vi "User Console.vi"(8 "error in":errorcluster) -> (0 "error out":errorcluster)   [LabVIEW 2020]
doc: "User Console thread VI"
uses:
  Controls/Events_User.ctl
  Database/Controls/Account Database.ctl
  Controls/Data_Initialize.ctl
  SubVIs/User Event - Stop/User Event - Stop.lvlib
  <vilib>/Utility/error.llb/Error Cluster From Error Code.vi
  <vilib>/ErrorRing/Error Ring.xnode
  SubVIs/Message Queue/Message Queue.lvlib
  SubVIs/Message Queue/Enqueue Message (Single).vi
  FGV/Controls/FGV_State.ctl
  Controls/User Console references.ctl
  Controls/User console Local Data.ctl
  Controls/Keypad.ctl
  Controls/Transactions.ctl
  Controls/User Console.ctl
panel:
  in  "User Console":T1
  # "[Covers: UI2]"
  # "[Covers: UI1]"
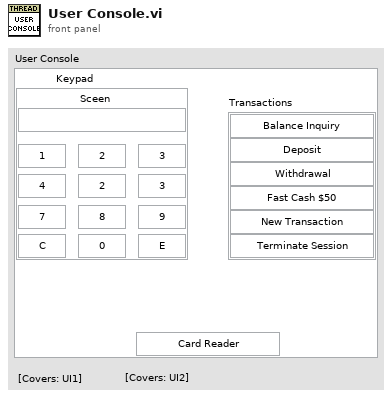
[diagram p1: front panel]
types:
  T1 = typedef "User Console.ctl" = cluster{"Keypad":T2, "Transactions":T3, "Card Reader":bool}
  T2 = typedef "Keypad.ctl" = cluster{"Sceen":string, "1":bool, "2":bool, "3":bool, "4":bool, "5":bool, "6":bool, "7":bool, "8":bool, "9":bool, "C":bool, "0":bool, "E":bool}
  T3 = typedef "Transactions.ctl" = cluster{"Balance Inquiry":bool, "Deposit":bool, "Withdrawal":bool, "Fast Cash $50":bool, "New Transaction":bool, "Terminate Session":bool}
  T4 = enum32{"Invalid", "Standard", "Closed", "Hidden", "Minimized", "Maximized"}
  T5 = typedef "FGV_State.ctl" = enum16{"1 - OpenDatabase", "2 - Initialize Events", "3 - Initialize QMH", "4 - Close QMH", "5 - Close Events", "Read FGV", "Save Database", "Def"}
  T6 = typedef "FGV_Data.ctl" = cluster{"QMH":T7, "User Events":T8, "Database":T9[]}
  T7 = typedef "Message Queue.lvlib/All Message Queues.ctl" = cluster{"User Console":refnum<queue>, "Display Console":refnum<queue>, "Sensor Interface":refnum<queue>, "Process":refnum<queue>}
  T8 = typedef "Events_User.ctl" = cluster{"Stop User Console":refnum<user-event>, "Error User Console":refnum<user-event>, "Stop Sensor Interface ":refnum<user-event>, "Error Sensor Interface":refnum<user-event>}
  T9 = typedef "Account Database.ctl" = cluster{"Account Number":i32, "First Name":string, "Last Name":string, "Balance":dbl}
  T10 = typedef "User console Local Data.ctl" = cluster{"Initiliaze":T11, "User Console Ref":T12, "Configuration Database":T9}
  T11 = typedef "Data_Initialize.ctl" = cluster{"Database":T9[], "User Events":T8}
  T12 = typedef "User Console references.ctl" = cluster{"0":refnum<vi>, "1":refnum<vi>, "2":refnum<vi>, "3":refnum<vi>, "4":refnum<vi>, "5":refnum<vi>, "6":refnum<vi>, "7":refnum<vi>, "8":refnum<vi>, "9":refnum<vi>, "Deposit":refnum<vi>, "Fast Cash $50":refnum<vi>, "Balance Inquiry":refnum<vi>, "Sceen":refnum<vi>, "Card Reader":refnum<vi>, "Withdrawal":refnum<vi>, "New Transaction":refnum<vi>, "Terminate Session":refnum<vi>, "E":refnum<vi>, "C":refnum<vi>}
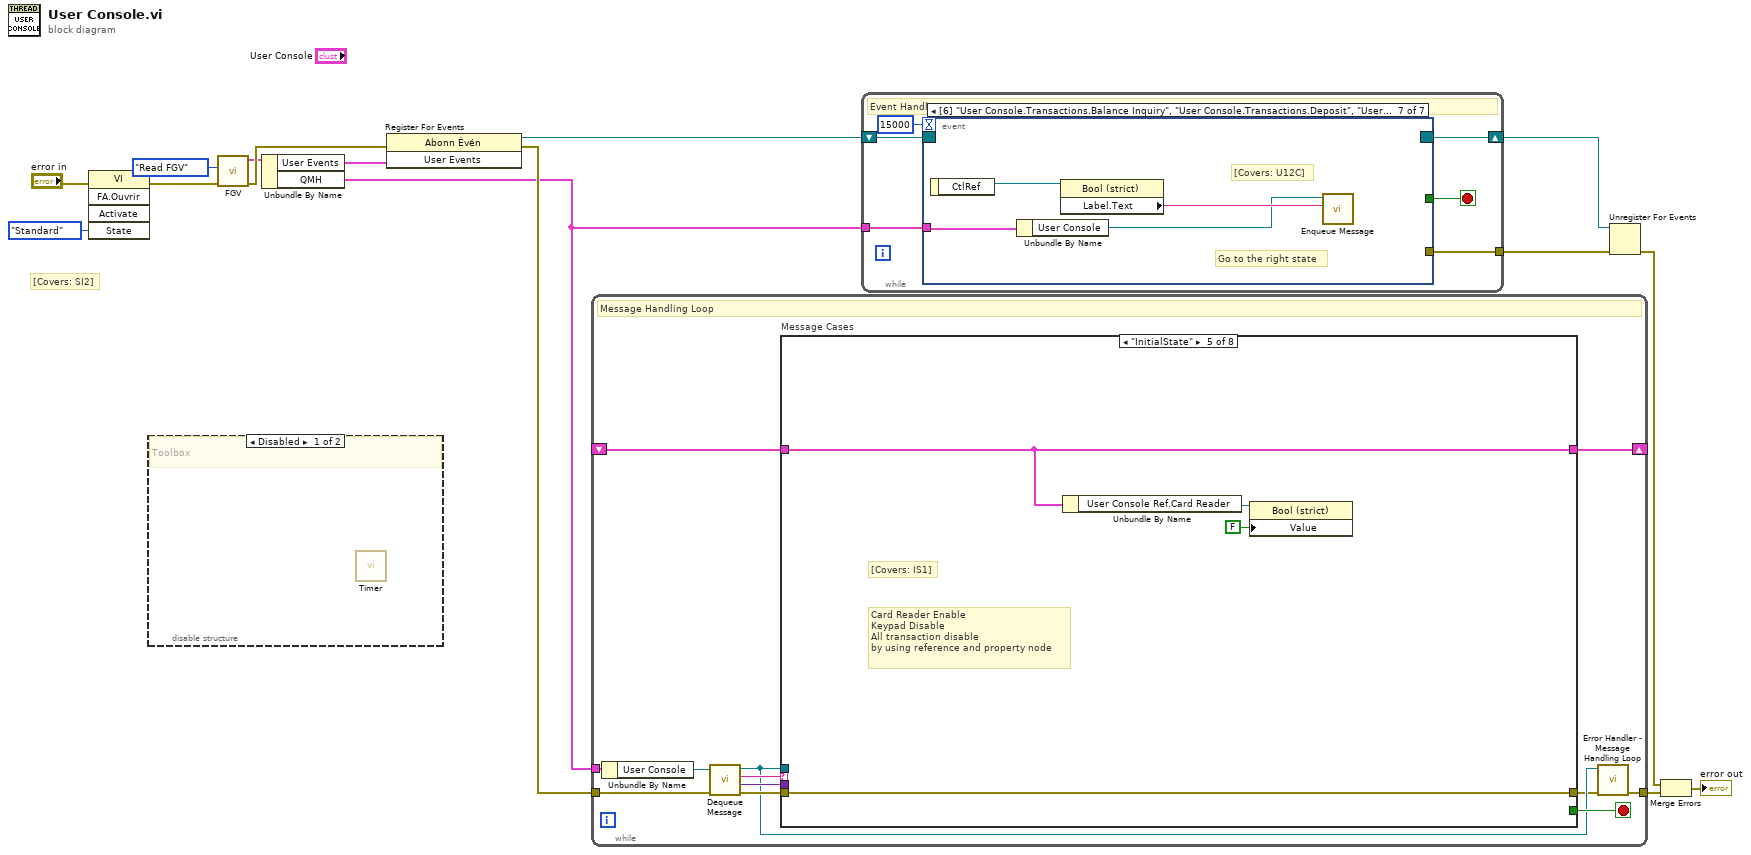
[diagram p0: block diagram]
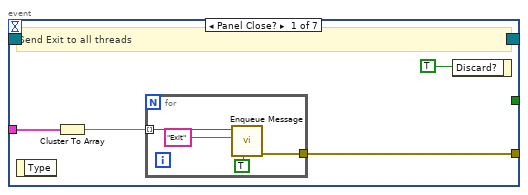
[diagram p3: hidden frame]
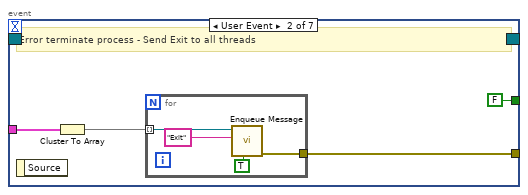
[diagram p4: hidden frame]
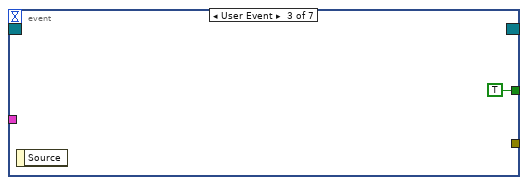
[diagram p5: hidden frame]
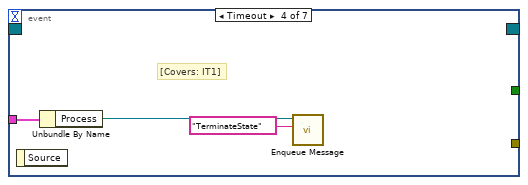
[diagram p6: hidden frame]
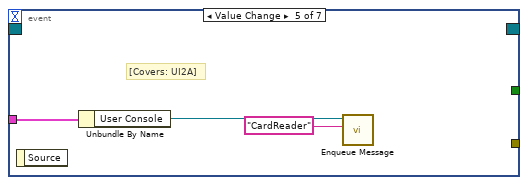
[diagram p7: hidden frame]
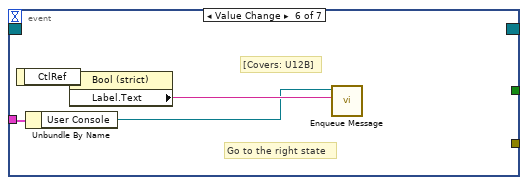
[diagram p8: hidden frame]
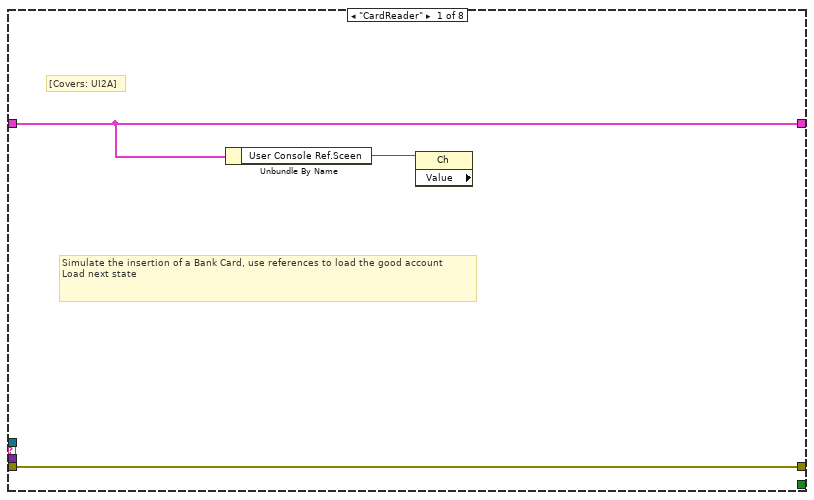
[diagram p9: hidden frame]
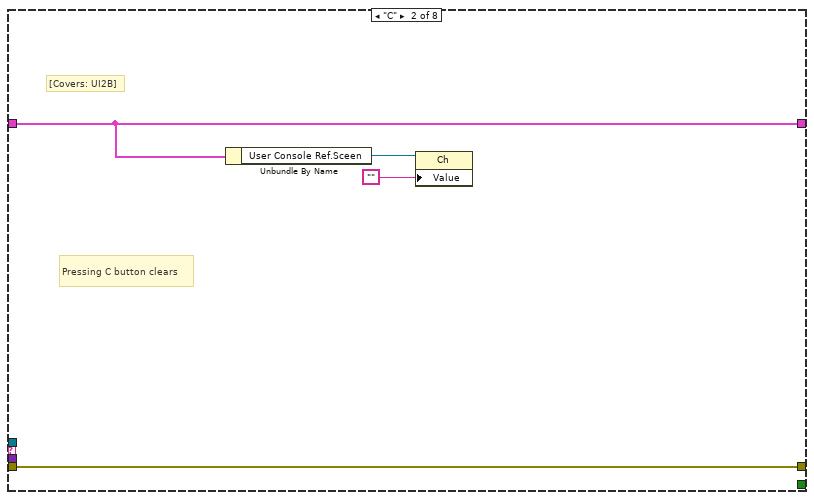
[diagram p10: hidden frame]
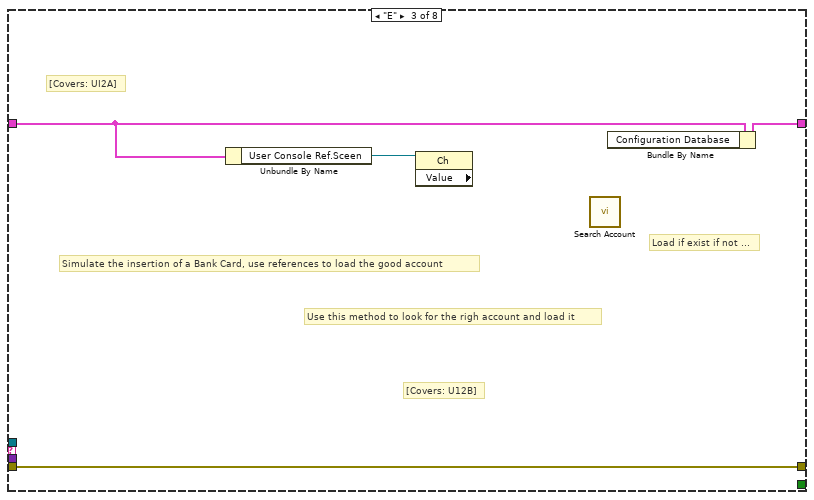
[diagram p11: hidden frame]
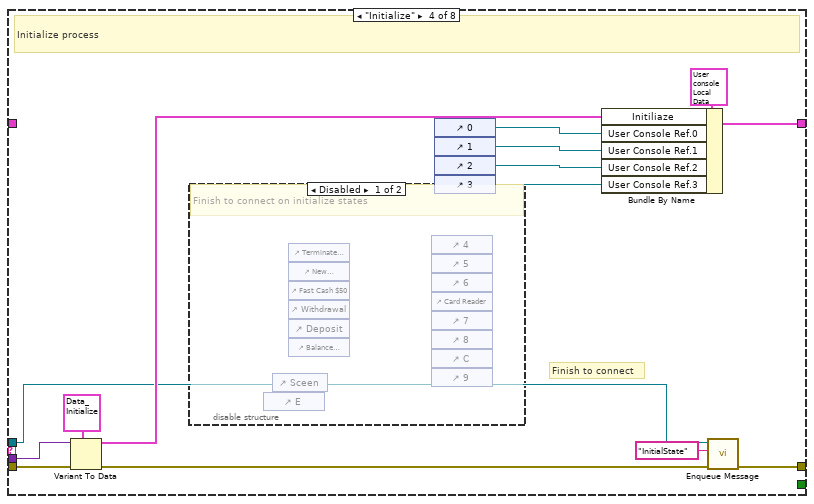
[diagram p12: hidden frame]
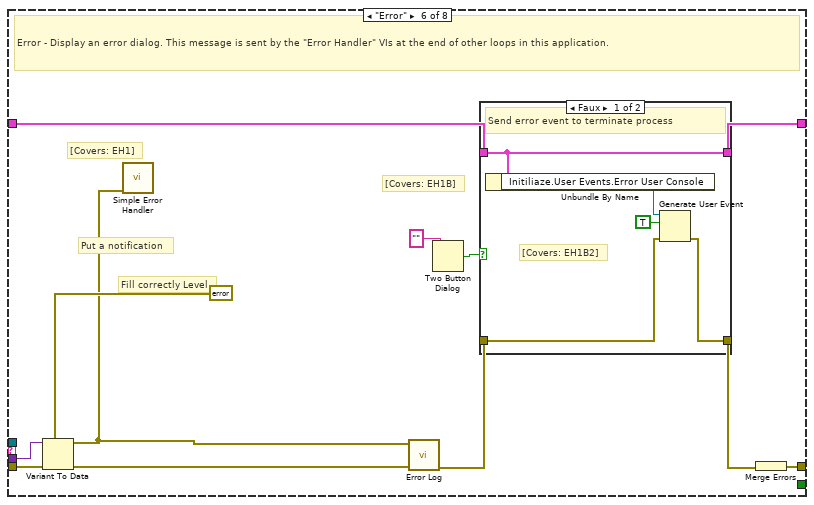
[diagram p14: hidden frame]
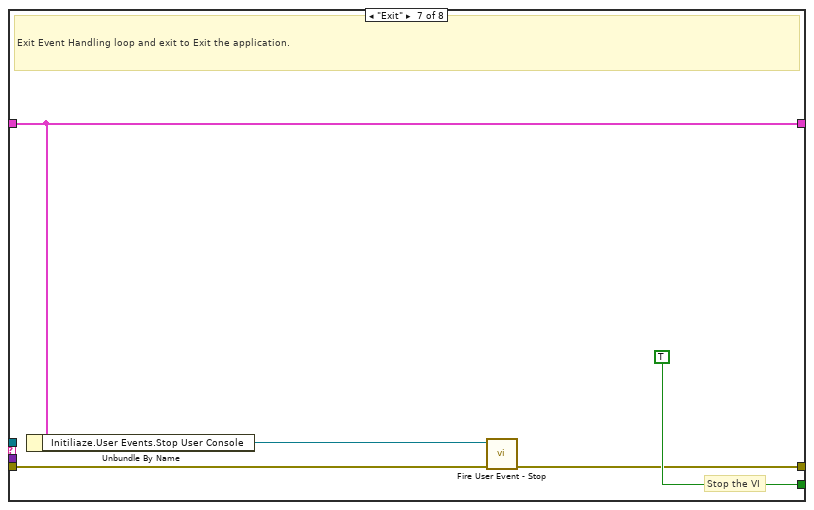
[diagram p16: hidden frame]
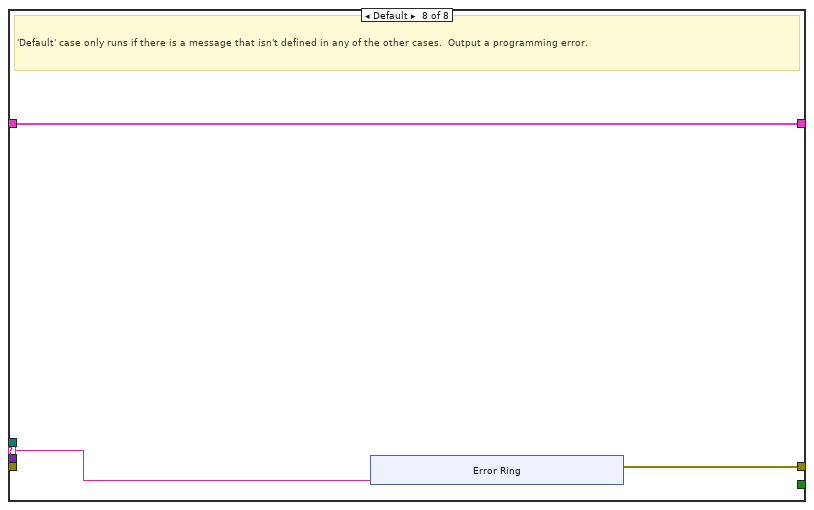
[diagram p17: hidden frame]
diagram:
  # "[Covers: SI2]"
  n1 = invoke class="VI" method="FA.Ouvrir"(error in="error in", "State"=T4."Standard") -> (error out=w2:errorcluster)  [unwired: 3 in, 4 out]
  n2 = disable-structure shown="Disabled" {
    frame Disabled {
      # "Toolbox"
      n3 = call "Timer.vi"() -> ()  [unwired: 9 in, 3 out]
    }
    frame Enabled {
    }
  }
  n4 = call "FGV.vi"("error in (no error)"=w2, "FGV_State"=FGV_State."Read FGV") -> ("error out"=w12:errorcluster, "FGV 2"=w10:T6)  [unwired: 8 in]
  n5 = Unbundle By Name(w10) -> ("User Events"=w11:T8, "QMH"=w14:T7)
  n6 = register-events(error in=w12, w11) -> (reference out=w8:refnum<event-registration>, error out=w15:errorcluster)  [unwired: 1 in]
  n7 = while {
    tunnel: w14 -> [w17]
    shift-right: [w26] -> _
    shift-left: _ -> [w27]
    tunnel: w15 -> [w24]
    tunnel: [w19] -> w4
    stop <- w25 stop-if-true
    # "Message Handling Loop"
    n8 = Unbundle By Name(w17) -> ("User Console"=w16:refnum<queue>)
    n9 = call "Dequeue Message.vi"("error in (no error)"=w24, "Message Queue"=w16) -> ("error out"=w23:errorcluster, "Message Data"=w21:variant, "Message"=w22:string, "dup Message Queue"=w20:refnum<queue>)  [unwired: 6 in]
    n10 = case "Message Cases" shown="\"InitialState\"" w22 {
      selector: w22 -> [_ _ _ _ _ _ _ w81]
      tunnel: w20 -> [_ _ _ w40 _ _ _ _]
      tunnel: w23 -> [w30 w34 w38 w51 w56 w68 w77 _]
      tunnel: [w30 w34 w38 w39 w56 w65 w76 w82] -> w18
      tunnel: w27 -> [w28 w32 w37 _ w55 w59 w79 w83]
      tunnel: [w28 w32 w35 w52 w55 w58 w79 w83] -> w26
      tunnel: [_ _ _ _ _ _ TRUE _] -> w25
      tunnel: w21 -> [_ _ _ w48 _ w67 _ _]
      frame "CardReader" {
        # "Simulate the insertion of a Bank Card, use references to load the good account\nLoad next state"
        # "[Covers: UI2A]"
        n11 = Unbundle By Name(w28) -> ("User Console Ref.Sceen"=w29:refnum<vi>)
        n12 = property class="Ch" props=["Value"](reference=w29) -> ()  [unwired: 1 in, 3 out]
      }
      frame "C" {
        # "Pressing C button clears"
        # "[Covers: UI2B]"
        n13 = Unbundle By Name(w32) -> ("User Console Ref.Sceen"=w33:refnum<vi>)
        n14 = property class="Ch"(reference=w33, "Value"="") -> ()  [unwired: 1 in, 2 out]
      }
      frame "E" {
        # "[Covers: U12B]"
        # "Load if exist if not ..."
        # "Use this method to look for the righ account and load it"
        # "Simulate the insertion of a Bank Card, use references to load the good account"
        # "[Covers: UI2A]"
        n15 = Unbundle By Name(w37) -> ("User Console Ref.Sceen"=w36:refnum<vi>)
        n16 = property class="Ch" props=["Value"](reference=w36) -> ()  [unwired: 1 in, 3 out]
        n17 = call "Search Account.vi"() -> ()  [unwired: 9 in, 3 out]
        n18 = Bundle By Name(cluster=w37) -> (w35:T10)  [unwired: 1 in]
      }
      frame "Initialize" {
        # "Finish to connect"
        # "Initialize process"
        n19 = Variant To Data(error in=w51, type=T11 {"Database"=[], "User Events"={"Stop User Console"=refnum, "Error User Console"=refnum, "Stop Sensor Interface "=refnum, "Error Sensor Interface"=refnum}} ("Initiliaze"), Variant=w48) -> (data=w49:T11, error out=w41:errorcluster)
        n20 = disable-structure shown="Disabled" {
          frame Disabled {
            # "Finish to connect on initialize states"
            n21 = control-ref of="E"() -> ()  [unwired: 1 out]
            n22 = control-ref of="Sceen"() -> ()  [unwired: 1 out]
            n23 = control-ref of="Terminate Session"() -> ()  [unwired: 1 out]
            n24 = control-ref of="New Transaction"() -> ()  [unwired: 1 out]
            n25 = control-ref of="Fast Cash $50"() -> ()  [unwired: 1 out]
            n26 = control-ref of="Withdrawal"() -> ()  [unwired: 1 out]
            n27 = control-ref of="Deposit"() -> ()  [unwired: 1 out]
            n28 = control-ref of="Balance Inquiry"() -> ()  [unwired: 1 out]
            n29 = control-ref of="4"() -> ()  [unwired: 1 out]
            n30 = control-ref of="5"() -> ()  [unwired: 1 out]
            n31 = control-ref of="6"() -> ()  [unwired: 1 out]
            n32 = control-ref of="Card Reader"() -> ()  [unwired: 1 out]
            n33 = control-ref of="7"() -> ()  [unwired: 1 out]
            n34 = control-ref of="8"() -> ()  [unwired: 1 out]
            n35 = control-ref of="C"() -> ()  [unwired: 1 out]
            n36 = control-ref of="9"() -> ()  [unwired: 1 out]
          }
          frame Enabled {
          }
        }
        n37 = control-ref of="0"() -> (w46:refnum<vi>)
        n38 = control-ref of="1"() -> (w45:refnum<vi>)
        n39 = control-ref of="2"() -> (w44:refnum<vi>)
        n40 = control-ref of="3"() -> (w43:refnum<vi>)
        n41 = Bundle By Name(cluster=T10 {"Initiliaze"={"Database"=[], "User Events"={"Stop User Console"=refnum, "Error User Console"=refnum, "Stop Sensor Interface "=refnum, "Error Sensor Interface"=refnum}}, "User Console Ref"={"0"=refnum, "1"=refnum, "2"=refnum, "3"=refnum, "4"=refnum, "5"=refnum, "6"=refnum, "7"=refnum, "8"=refnum, "9"=refnum, "Deposit"=refnum, "Fast Cash $50"=refnum, "Balance Inquiry"=refnum, "Sceen"=refnum, "Card Reader"=refnum, "Withdrawal"=refnum, "New Transaction"=refnum, "Terminate Session"=refnum, "E"=refnum, "C"=refnum}, "Configuration Database"={"Account Number"=0, "First Name"="", "Last Name"="", "Balance"=0.0}} ("Local Data"), "Initiliaze"=w49, "User Console Ref.0"=w46, "User Console Ref.1"=w45, "User Console Ref.2"=w44, "User Console Ref.3"=w43) -> (w52:T10)
        n42 = call-poly "Enqueue Message.vi"("error in (no error)"=w41, "Message"="InitialState", "Message Queue"=w40) -> ("error out"=w39:errorcluster)  [unwired: 7 in, 1 out]
      }
      frame "InitialState" {
        # "Card Reader Enable\nKeypad Disable\nAll transaction disable\nby using reference and property node"
        # "[Covers: IS1]"
        n43 = Unbundle By Name(w55) -> ("User Console Ref.Card Reader"=w54:refnum<vi>)
        n44 = property class="Bool (strict)"(reference=w54, "Value"=FALSE) -> ()  [unwired: 1 in, 2 out]
      }
      frame "Error" {
        # "Put a notification"
        # "[Covers: EH1B]"
        # "[Covers: EH1]"
        # "Fill correctly Level"
        # "Error - Display an error dialog. This message is sent by the \"Error Handler\" VIs at the end of other loops in this application."
        n45 = Variant To Data(error in=w68, type=errorcluster {"status"=FALSE, "code"=0, "source"=""} ("error constant"), Variant=w67) -> (data=w63:errorcluster, error out=w64:errorcluster)
        n46 = call <vilib>:"Simple Error Handler.vi"("error in (no error)"=w63) -> ()  [unwired: 4 in, 5 out]
        n47 = call "Error Log.vi"("error in"=w64, "error happened"=w63) -> ("error out"=w62:errorcluster)  [unwired: 9 in]
        n48 = Two Button Dialog(message="") -> (T button?=w61:bool)  [unwired: 2 in]
        n49 = case shown="Faux" w61 {
          tunnel: w62 -> [w71 w75]
          tunnel: [w70 w75] -> w60
          tunnel: w59 -> [w73 w74]
          tunnel: [w73 w74] -> w58
          frame False {
            # "[Covers: EH1B2]"
            # "Send error event to terminate process"
            n50 = Unbundle By Name(w73) -> ("Initiliaze.User Events.Error User Console"=w72:refnum<user-event>)
            n51 = Generate User Event(user event=w72, event data cluster=TRUE ("event data"), error in=w71) -> (error out=w70:errorcluster)  [unwired: 1 in, 1 out]
          }
          frame True {
            # "[Covers: EH1B1]"
            # "Continu (ok)"
          }
        }
        n52 = Merge Errors(w60) -> (w65:errorcluster)
      }
      frame "Exit" {
        # "Stop the VI"
        # "Exit Event Handling loop and exit to Exit the application."
        n53 = Unbundle By Name(w79) -> ("Initiliaze.User Events.Stop User Console"=w78:refnum<user-event>)
        n54 = call "Fire User Event - Stop.vi"("error in (no error)"=w77, "User Event - Stop"=w78) -> ("error out"=w76:errorcluster)  [unwired: 9 in]
      }
      frame Default {
        # "'Default' case only runs if there is a message that isn't defined in any of the other cases.  Output a programming error."
        n55 = xnode "Error Ring"("paramètre 0"=w81) -> ("sortie d'erreur"=w82:errorcluster)
      }
    }
    n56 = call "Error Handler - Message Handling Loop.vi"("error in (no error)"=w18, "Message Queue"=w20) -> ("dup error in"=w19:errorcluster)  [unwired: 8 in, 1 out]
  }
  n57 = while {
    tunnel: w14 -> [w96]
    shift-right: [w94] -> w6
    shift-left: w8 -> [w95]
    tunnel: [w92] -> w7
    stop <- w93 stop-if-true
    # "Event Handling Loop"
    n58 = event shown="[6] \"User Console.Transactions.Balance Inquiry\", \"User Console.Transactions.Deposit\", \"User Console.Transactions.Withdrawal\", \"User Console.Transactions.Fast Cash $50\", \"User Console.Transactions.New Transaction\", \"User Console.Transactions.Terminate Session\": Valeur changée" {
      selector: w95 -> [_ _ _ _ _ _ _]
      dyn-events: [_ _ _ _ _ _ _] -> w94
      timeout: 15000 -> [_ _ _ _ _ _ _]
      tunnel: [_ FALSE ("Discard?") TRUE ("Discard?") _ _ _ _] -> w93
      tunnel: w96 -> [w99 w108 _ w115 w117 w121 w124]
      tunnel: [w98 w107 _ _ _ _ _] -> w92
      event Panel Close? {
        # "Send Exit to all threads"
        n59 = event-data() -> ()  [unwired: 1 in, 1 out]
        n60 = Cluster To Array(cluster=w99) -> (array=w97:refnum<queue>[])
        n61 = for {
          tunnel: w97 -> [w104] mode=indexing
          tunnel: [w103] -> w98
          n62 = call-poly "Enqueue Message.vi"("Priority Message? (F)"=TRUE, "Message"="Exit", "Message Queue"=w104) -> ("error out"=w103:errorcluster)  [unwired: 7 in, 1 out]
        }
        n63 = event-data("Discard?"=TRUE) -> ()  [unwired: 1 in, 1 out]
      }
      event User Event {
        # "Error terminate process - Send Exit to all threads"
        n64 = event-data() -> ()  [unwired: 1 in, 1 out]
        n65 = Cluster To Array(cluster=w108) -> (array=w106:refnum<queue>[])
        n66 = for {
          tunnel: w106 -> [w112] mode=indexing
          tunnel: [w111] -> w107
          n67 = call-poly "Enqueue Message.vi"("Priority Message? (F)"=TRUE, "Message"="Exit", "Message Queue"=w112) -> ("error out"=w111:errorcluster)  [unwired: 7 in, 1 out]
        }
      }
      event User Event {
        n68 = event-data() -> ()  [unwired: 1 in, 1 out]
      }
      event Timeout {
        # "[Covers: IT1]"
        n69 = event-data() -> ()  [unwired: 1 in, 1 out]
        n70 = Unbundle By Name(w115) -> ("Process"=w114:refnum<queue>)
        n71 = call-poly "Enqueue Message.vi"("Message"="TerminateState", "Message Queue"=w114) -> ()  [unwired: 8 in, 2 out]
      }
      event Value Change {
        # "[Covers: UI2A]"
        n72 = event-data() -> ()  [unwired: 1 in, 1 out]
        n73 = Unbundle By Name(w117) -> ("User Console"=w118:refnum<queue>)
        n74 = call-poly "Enqueue Message.vi"("Message"="CardReader", "Message Queue"=w118) -> ()  [unwired: 8 in, 2 out]
      }
      event Value Change {
        # "[Covers: U12B]"
        # "Go to the right state"
        n75 = event-data() -> ("CtlRef"=w123:refnum<vi>)  [unwired: 1 in]
        n76 = Unbundle By Name(w121) -> ("User Console"=w120:refnum<queue>)
        n77 = property class="Bool (strict)"(reference=w123) -> ("Label.Text"=w122:string)  [unwired: 1 in, 2 out]
        n78 = call-poly "Enqueue Message.vi"("Message"=w122, "Message Queue"=w120) -> ()  [unwired: 8 in, 2 out]
      }
      event Value Change {
        # "[Covers: U12C]"
        # "Go to the right state"
        n79 = event-data() -> ("CtlRef"=w125:refnum<vi>)  [unwired: 1 in]
        n80 = Unbundle By Name(w124) -> ("User Console"=w126:refnum<queue>)
        n81 = property class="Bool (strict)"(reference=w125) -> ("Label.Text"=w127:string)  [unwired: 1 in, 2 out]
        n82 = call-poly "Enqueue Message.vi"("Message"=w127, "Message Queue"=w126) -> ()  [unwired: 8 in, 2 out]
      }
    }
  }
  n83 = Unregister For Events(event registration refnum=w6, error in=w7) -> (error out=w5:errorcluster)
  n84 = Merge Errors(w5, w4) -> (→"error out":errorcluster)
